vi "Target Motor Current Rate Limiter.vi"(8 "Max Negative Difference":dbl, 9 "Max Positive Difference":dbl, 11 "Motor Command":dbl) -> (2 "Filtered Motor Command":dbl)   [LabVIEW 2018]
panel:
  out "Previous Filtered Motor Command":dbl
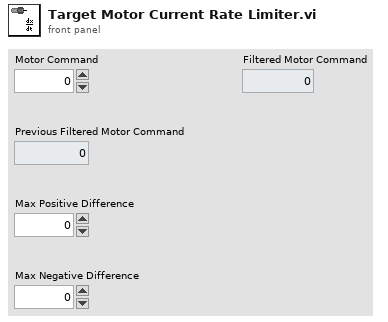
[diagram p1: front panel]
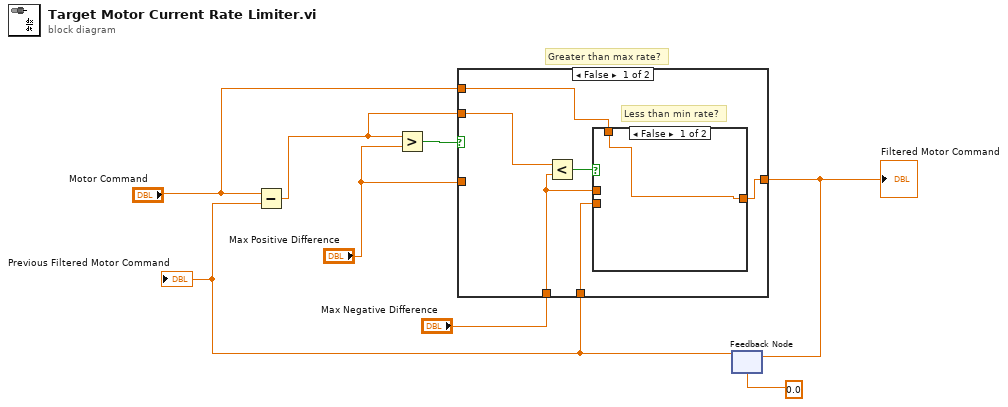
[diagram p0: block diagram]
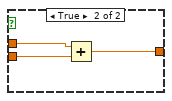
[diagram p2: hidden frame]
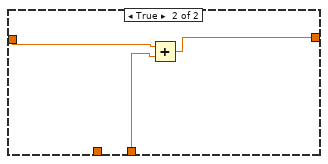
[diagram p3: hidden frame]
diagram:
  # "Greater than max rate?"
  n1 = feedback #1(0.0 ("Motor Command")) -> (w5:dbl)
  "Previous Filtered Motor Command" <- w5
  n2 = Subtract(x="Motor Command", y=w5) -> (x-y=w3:dbl)
  n3 = Greater?(x=w3, y="Max Positive Difference") -> (0:w8:bool)
  n4 = case shown="False" w8 {
    tunnel: w5 -> [w13 w21]
    tunnel: [w11 w20] -> w6
    tunnel: "Max Positive Difference" -> [_ w19]
    tunnel: w3 -> [w10 _]
    tunnel: "Max Negative Difference" -> [w12 _]
    tunnel: "Motor Command" -> [w9 _]
    frame False {
      # "Less than min rate?"
      n5 = Less?(x=w10, y=w12) -> (x < y?=w14:bool)
      n6 = case shown="False" w14 {
        tunnel: w13 -> [_ w18]
        tunnel: w12 -> [_ w17]
        tunnel: [w15 w16] -> w11
        tunnel: w9 -> [w15 _]
        frame False {
        }
        frame True {
          n7 = Add(x=w17, y=w18) -> (x+y=w16:dbl)
        }
      }
    }
    frame True {
      n8 = Add(x=w19, y=w21) -> (x+y=w20:dbl)
    }
  }
  "Filtered Motor Command" <- w6
  n9 = feedback-in #1(w6) -> ()
